vi "Read (No Check) U16.vi"(8 "error in (no error)":errorcluster, 9 "offset (0)":u64 format="%d bytes", 10 "value in":u16, 11 "Pointer in":refnum<class "Pointer.lvclass">) -> (0 "error out":errorcluster, 1 "offset + size":u64 format="%d bytes", 2 "value out":u16, 3 "Pointer out":refnum<class "Pointer.lvclass">)   [LabVIEW 2020, in "Memory Manager.lvlib" / "Pointer.lvclass"]
doc: "Reads <b>value</b> from the address specified by <b>pointer + offset</b>.\n\n<b>Note:</b> This VI is <b>unsafe</b>.\n\nUnsafe means that it does not evaluate the size parameter of <b>pointer</b> to ensure that is inbounds of allocated memory before peforming a memory read/write. Reading/writing more data to a pointer than it has allocated can corrupt or crash LabVIEW. Only use this VI in scenarios where the <b>pointer</b> has been validated to be allocated to a correct size before calling this VI."
uses:
  Pointer.lvclass
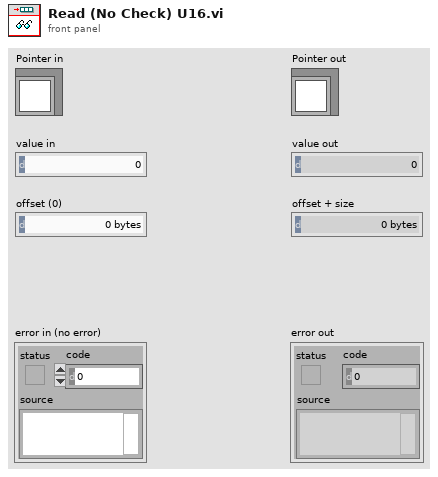
[diagram p1: front panel]
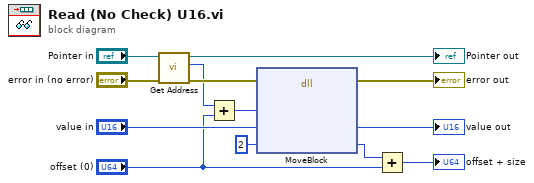
[diagram p0: block diagram]
diagram:
  n1 = call "Get Address.vi"("Pointer in"="Pointer in") -> ("address"=w4:u64, "Pointer out"=→"Pointer out":refnum<class "Pointer.lvclass">)  [unwired: 9 in]
  n2 = Add(x=w4, y="offset (0)") -> (x+y=w6:u64)
  n3 = dll-call lib="LabVIEW" fn="MoveBlock"(error in="error in (no error)", "src"=w6, "dst"="value in", "size"=u64 2) -> (error out=→"error out":errorcluster, "dst"=→"value out":u16, "size"=w1:u64)  [unwired: 4 in, 1 out]
  n4 = Add(x=w1, y="offset (0)") -> (x+y=→"offset + size":u64)
